vi "Read Configuration from File.vi"(8 "Error In":errorcluster, 10 "Configuration File Path":path=path "C:/CSPP-RT.ini", 11 "CS++RTWatchdogActor in":refnum<class "CS++RTWatchdogActor.lvclass">) -> (0 "Error Out":errorcluster, 3 "CS++RTWatchdogActor out":refnum<class "CS++RTWatchdogActor.lvclass">)   [LabVIEW 2014, in "CS++RTWatchdog.lvlib" / "CS++RTWatchdogActor.lvclass"]
doc: "Read watchdog configuration from ini-file."
uses:
  CS++RTWatchdogActor.lvclass
  CS++RTWatchdogActor.lvclass/CS++RTWatchdogActor.ctl
  <vilib>/Utility/config.llb/Read Key (Boolean).vi
  <vilib>/Utility/config.llb/Read Key (I32).vi
  <vilib>/Utility/config.llb/Read Key (Double).vi
  <vilib>/Utility/config.llb/NI_LVConfig.lvlib
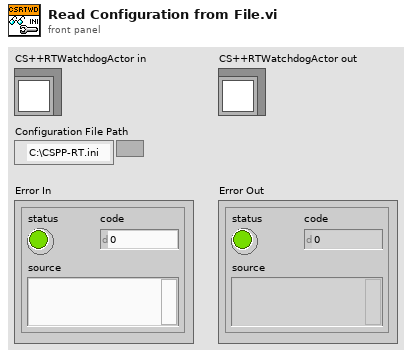
[diagram p1: front panel]
types:
  T1 = enum16{"active high", "active low", "open collector"}
  T2 = enum16{"none", "line 0", "line 1", "line 2", "line 3", "line 4", "line 5", "line 6", "line 7", "SMB line 0"}
  T3 = typedef "NI_LVConfig.lvlib/Config Data RefNum.ctl" = refnum<k1>
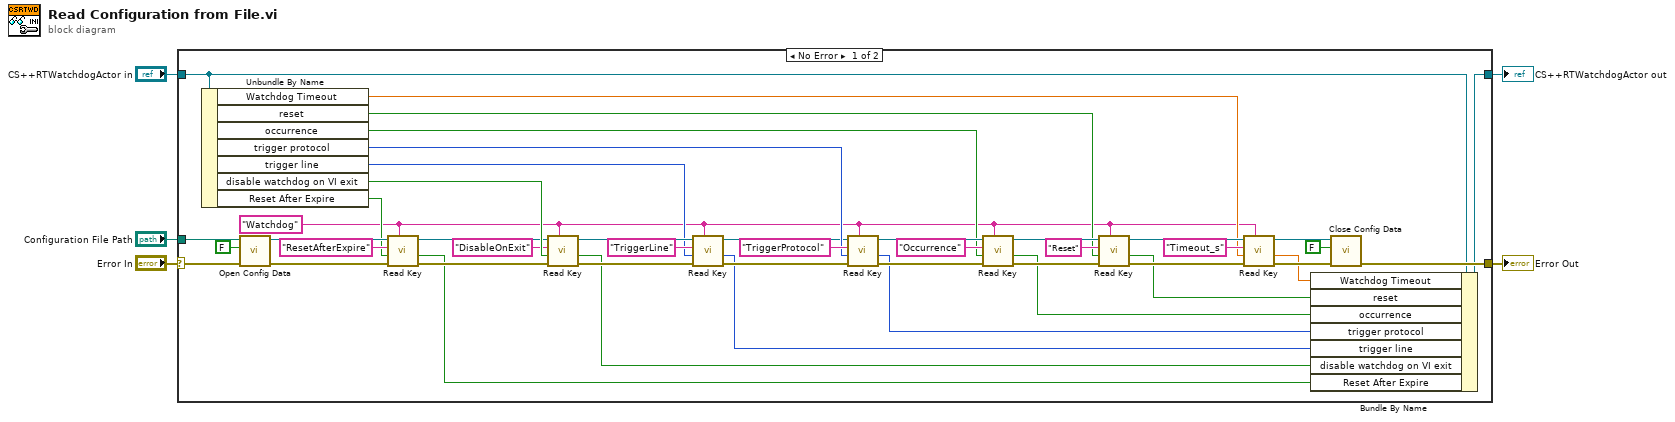
[diagram p0: block diagram]
diagram:
  n1 = case shown="No Error" "Error In" {
    selector: "Error In" -> [w50 w52]
    tunnel: [w25 w52] -> w4
    tunnel: [w19 w51] -> w2
    tunnel: "CS++RTWatchdogActor in" -> [w20 w51]
    tunnel: "Configuration File Path" -> [w49 _]
    frame No Error {
      w6 = "Watchdog" ("section")
      n2 = Unbundle By Name(w20) -> ("Watchdog Timeout"=w26:dbl, "reset"=w30:bool, "occurrence"=w34:bool, "trigger protocol"=w40:T1, "trigger line"=w42:T2, "disable watchdog on VI exit"=w47:bool, "Reset After Expire"=w8:bool)
      n3 = call <vilib>:"Open Config Data.vi"("error in (no error)"=w50, "create file if necessary (T)"=FALSE, "configuration file path"=w49) -> ("error out"=w9:errorcluster, "refnum"=w12:T3)  [unwired: 6 in, 1 out]
      n4 = call-poly <vilib>:"Read Key.vi"("section"=w6, "error in (no error)"=w9, "default value"=w8, "key"="ResetAfterExpire", "refnum"=w12) -> ("error out"=w10:errorcluster, "value"=w7:bool, "refnum out"=w11:T3)  [unwired: 3 in, 1 out]
      n5 = call-poly <vilib>:"Read Key.vi"("section"=w6, "error in (no error)"=w10, "default value"=w47, "key"="DisableOnExit", "refnum"=w11) -> ("error out"=w44:errorcluster, "value"=w14:bool, "refnum out"=w45:T3)  [unwired: 3 in, 1 out]
      n6 = call-poly <vilib>:"Read Key.vi"("section"=w6, "error in (no error)"=w44, "default value"=w42, "key"="TriggerLine", "refnum"=w45) -> ("error out"=w39:errorcluster, "value"=w15:i32, "refnum out"=w38:T3)  [unwired: 3 in, 1 out]
      n7 = call-poly <vilib>:"Read Key.vi"("section"=w6, "error in (no error)"=w39, "default value"=w40, "key"="TriggerProtocol", "refnum"=w38) -> ("error out"=w35:errorcluster, "value"=w16:i32, "refnum out"=w36:T3)  [unwired: 3 in, 1 out]
      n8 = call-poly <vilib>:"Read Key.vi"("section"=w6, "error in (no error)"=w35, "default value"=w34, "key"="Occurrence", "refnum"=w36) -> ("error out"=w31:errorcluster, "value"=w17:bool, "refnum out"=w32:T3)  [unwired: 3 in, 1 out]
      n9 = call-poly <vilib>:"Read Key.vi"("section"=w6, "error in (no error)"=w31, "default value"=w30, "key"="Reset", "refnum"=w32) -> ("error out"=w27:errorcluster, "value"=w18:bool, "refnum out"=w28:T3)  [unwired: 3 in, 1 out]
      n10 = call-poly <vilib>:"Read Key.vi"("section"=w6, "error in (no error)"=w27, "default value"=w26, "key"="Timeout_s", "refnum"=w28) -> ("error out"=w23:errorcluster, "value"=w21:dbl, "refnum out"=w24:T3)  [unwired: 3 in, 1 out]
      n11 = Bundle By Name(cluster=w20, "Watchdog Timeout"=w21, "reset"=w18, "occurrence"=w17, "trigger protocol"=w16, "trigger line"=w15, "disable watchdog on VI exit"=w14, "Reset After Expire"=w7) -> (w19:refnum<class "CS++RTWatchdogActor.lvclass">)
      n12 = call <vilib>:"Close Config Data.vi"("error in (no error)"=w23, "write file if changed (T)"=FALSE, "refnum"=w24) -> ("error out"=w25:errorcluster)  [unwired: 7 in, 1 out]
    }
    frame Error {
    }
  }
  "Error Out" <- w4
  "CS++RTWatchdogActor out" <- w2
